vi "ExampleCodeModule.vi"(9 "CurrentAllowBreakStationSetting":bool, 10 "UseExternallySuspended":bool, 11 "Sequence Context":refnum<k7>) -> (0 "error out":errorcluster)   [LabVIEW 2011]
uses:
  ExecStates.ctl
panel:
  out "TestStand Execution Status":T1
  out "Test Simulation":dbl(graph)
  in  "OK":bool
  # "By default, A TestStand execution cannot be paused, such as at a breakpoint if one or more threads in the execution are running a code module.\n\nHowever, if one or both of the options below are enabled, the execution will be able to break even if the thread is running a code module.  This code module polls the execution status and pauses testing if the TestStand execution is suspended."
  # "Current Configuration"
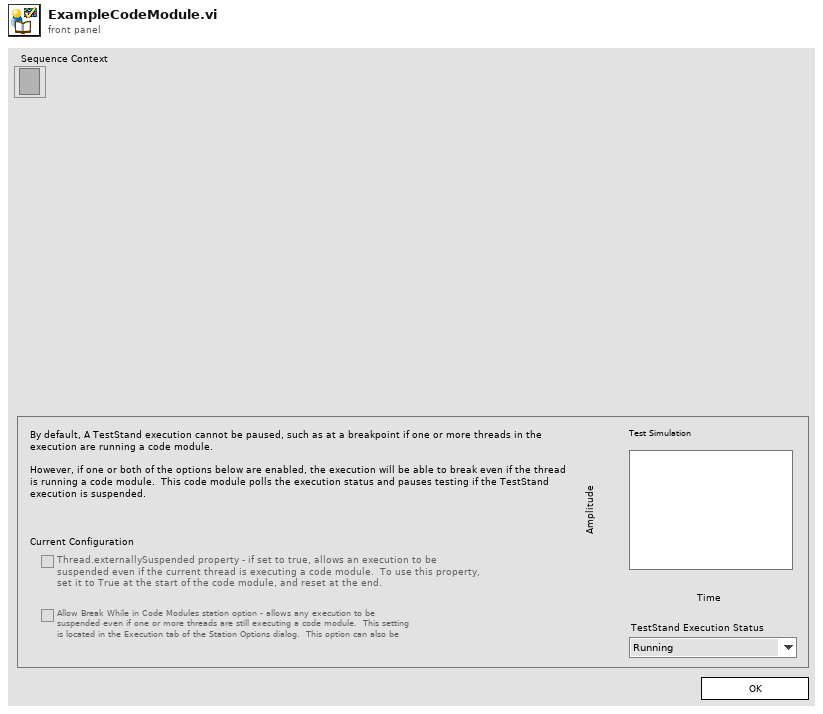
[diagram p1: front panel]
types:
  T1 = typedef "ExecStates.ctl" = enum16{"Running", "Paused"}
  T2 = typedef "TestStand - Status Monitor.ctl" = cluster{"Sequence Context":refnum<k7>, "Execution":refnum<k7>, "Termination Monitor":refnum<k7>}
  T3 = enum8{"Enabled", "Disabled", "Disabled and Grayed Out"}
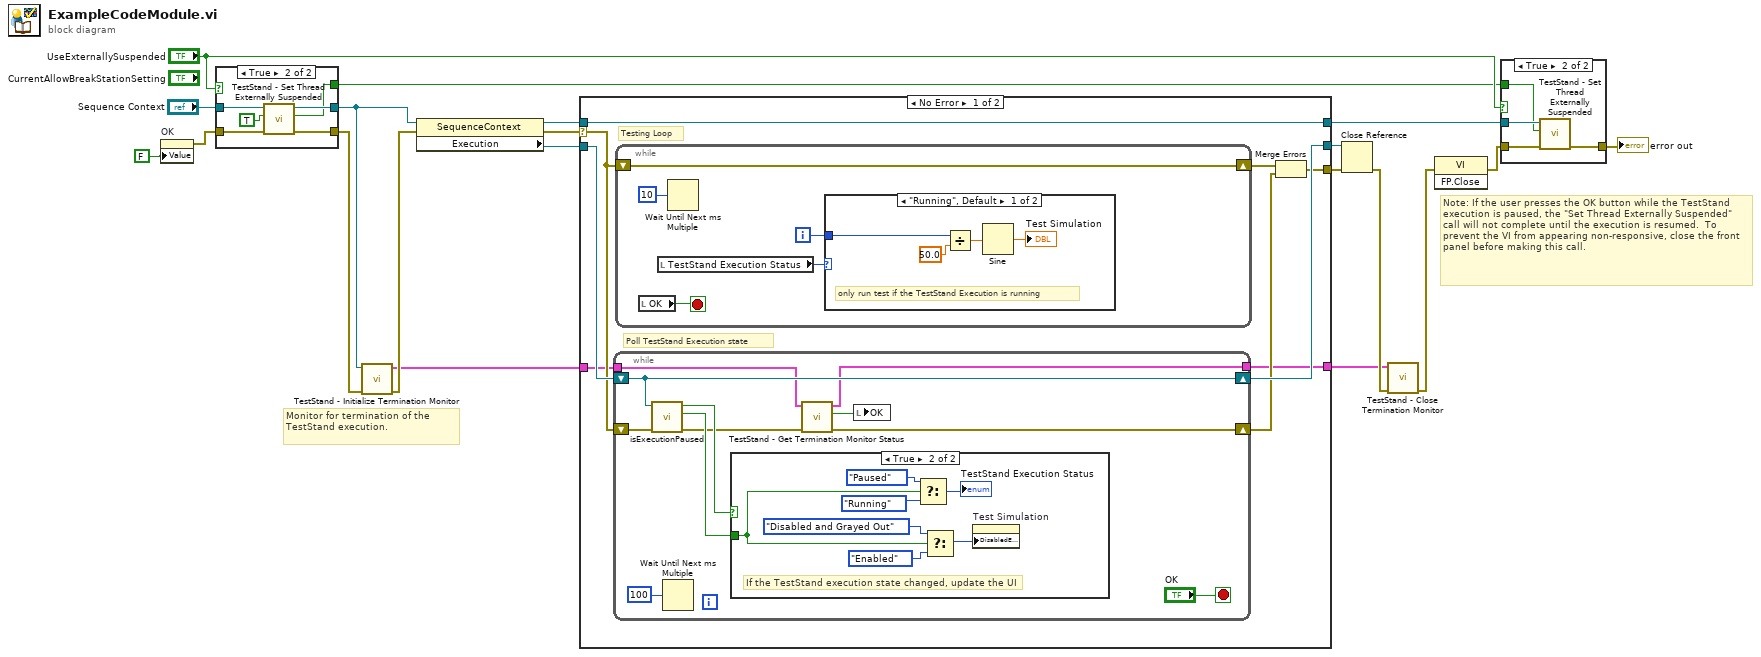
[diagram p0: block diagram]
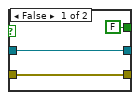
[diagram p3: hidden frame]
diagram:
  # "Monitor for termination of the TestStand execution."
  # "Note: If the user presses the OK button while the TestStand execution is paused, the \"Set Thread Externally Suspended\" call will not complete until the execution is resumed.  To prevent the VI from appearing non-responsive, close the front panel before making this call."
  n1 = property on="OK" class="Bool (strict)"("Value"=FALSE ("OK")) -> (error out=w9:errorcluster)  [unwired: 2 in, 1 out]
  n2 = case shown="True" "UseExternallySuspended" {
    tunnel: [w22 w29] -> w7
    tunnel: "Sequence Context" -> [w23 w28]
    tunnel: [w23 w27] -> w5
    tunnel: w9 -> [w22 w25]
    tunnel: [FALSE ("Previous Externally Suspended") w24] -> w1
    frame False {
    }
    frame True {
      n3 = call <vilib>:"TestStand - Set Thread Externally Suspended.vi"("error in (no error)"=w25, "Externally Suspended (T)"=TRUE, "Sequence Context In"=w28) -> ("error out"=w29:errorcluster, "Previous Externally Suspended"=w24:bool, "Sequence Context Out"=w27:refnum<k7>)  [unwired: 2 in]
    }
  }
  n4 = call <vilib>:"TestStand - Initialize Termination Monitor.vi"("error in (no error)"=w7, "Sequence Context In"=w5) -> ("error out"=w8:errorcluster, "Status Monitor Out"=w6:T2)  [unwired: 8 in]
  n5 = property class="SequenceContext"(reference=w5, error in=w8) -> (reference out=w16:refnum<k7>, error out=w14:errorcluster, "Execution"=w18:refnum<k7>)
  n6 = case shown="No Error" w14 {
    selector: w14 -> [w35 w67]
    tunnel: [w38 w69] -> w20
    tunnel: w16 -> [w38 w69]
    tunnel: w18 -> [w37 w68]
    tunnel: [w36 w68] -> w15
    tunnel: [w34 w67] -> w13
    tunnel: w6 -> [w31 w66]
    tunnel: [w30 w66] -> w3
    frame No Error {
      # "Poll TestStand Execution state"
      # "Testing Loop"
      n7 = while {
        shift-right: [w57] -> w36
        shift-left: w37 -> [w57]
        shift-right: [w50] -> w33
        shift-left: w35 -> [w54]
        tunnel: w31 -> [w53]
        tunnel: [w52] -> w30
        stop <- "OK" stop-if-true
        n8 = call "isExecutionPaused.vi"("error in (no error)"=w54, "Execution"=w57) -> ("error out"=w51:errorcluster, "Execution Paused"=w56:bool, "State Changed"=w55:bool)  [unwired: 7 in]
        n9 = Wait Until Next ms Multiple(millisecond multiple=u32 100) -> ()  [unwired: 1 out]
        n10 = case shown="True" w55 {
          tunnel: w56 -> [_ w63]
          frame False {
          }
          frame True {
            # "If the TestStand execution state changed, update the UI"
            n11 = Select(t=ExecStates."Paused" ("Execution Status"), s=w63, f=ExecStates."Running" ("Execution Status")) -> (s? t:f=→"TestStand Execution Status":T1)
            n12 = Select(t=T3."Disabled and Grayed Out" ("Disabled"), s=w63, f=T3."Enabled" ("Disabled")) -> (s? t:f=w61:T3)
            n13 = property on="Test Simulation" class="WFChart (strict)"("DisabledEnum"=w61) -> ()  [unwired: 2 in, 2 out]
          }
        }
        n14 = call <vilib>:"TestStand - Get Termination Monitor Status.vi"("error in (no error)"=w51, "Status Monitor In"=w53) -> ("error out"=w50:errorcluster, "Terminating or Aborting"=w48:bool, "Status Monitor Out"=w52:T2)  [unwired: 7 in]
        n15 = local write "OK"(w48) -> ()
      }
      n16 = while {
        shift-right: [w41] -> w32
        shift-left: w35 -> [w41]
        i -> [w42]
        stop <- w40 stop-if-true
        n17 = local read "OK"() -> (w40:bool)
        n18 = local read "TestStand Execution Status"() -> (w39:T1)
        n19 = Wait Until Next ms Multiple(millisecond multiple=u32 10) -> ()  [unwired: 1 out]
        n20 = case shown="\"Running\", Default" w39 {
          tunnel: w42 -> [w46 _]
          frame "Running", Default {
            # "only run test if the TestStand Execution is running"
            n21 = Divide(x=w46, y=50.0) -> (x/y=w44:dbl)
            n22 = Sine(x=w44) -> (sin(x)=→"Test Simulation":dbl)
          }
          frame "Paused" {
          }
        }
      }
      n23 = Merge Errors(w32, w33) -> (w34:errorcluster)
    }
    frame Error {
    }
  }
  n24 = Close Reference(reference=w15, error in (no error)=w13) -> (error out=w4:errorcluster)
  n25 = call <vilib>:"TestStand - Close Termination Monitor.vi"("error in (no error)"=w4, "Status Monitor In"=w3) -> ("error out"=w2:errorcluster)  [unwired: 9 in]
  n26 = invoke class="VI" method="FP.Close"(error in=w2) -> (error out=w11:errorcluster)  [unwired: 2 in, 2 out]
  n27 = case shown="True" "UseExternallySuspended" {
    tunnel: w11 -> [w70 w74]
    tunnel: [w70 w73] -> w12
    tunnel: w20 -> [_ w72]
    tunnel: w1 -> [_ w71]
    frame False {
    }
    frame True {
      n28 = call <vilib>:"TestStand - Set Thread Externally Suspended.vi"("error in (no error)"=w74, "Externally Suspended (T)"=w71, "Sequence Context In"=w72) -> ("error out"=w73:errorcluster)  [unwired: 2 in, 2 out]
    }
  }
  "error out" <- w12
